vi "Validate File Path.vi"(0 "File Path":path, 1 "Check Exist (F)":bool, 2 "Type":string, 3 "Error In":errorcluster, 4 "Check Type (F)":bool) -> (5 "Valid":bool, 6 "Error Out":errorcluster)   [LabVIEW 2018]
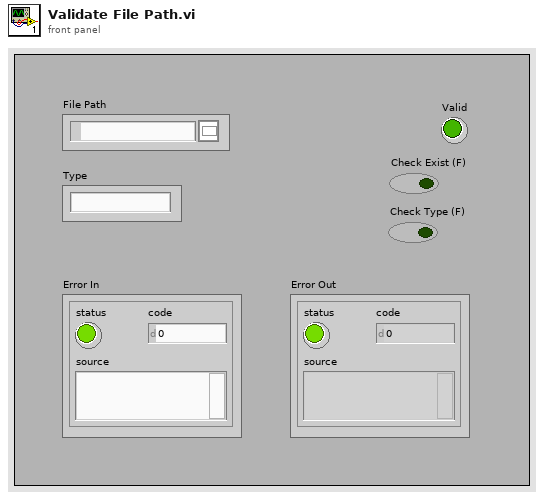
[diagram p1: front panel]
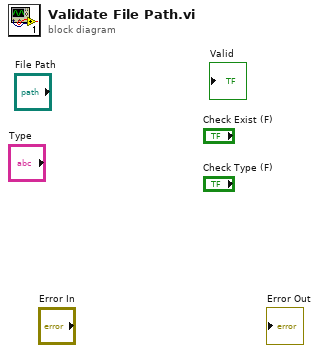
[diagram p0: block diagram]
diagram:
